vi "APC_9056_StateMachine.vi"(0 "ManualState":i8, 4 "ForceState":bool, 5 "PC_ControlSettings":T1={"Spark advance [CADBTDC]"=0.0, "Pref"=0.0, "O2ref"=0.0, "DI advance [CADBTDC]"=0.0, "DI duration [ms] "=0.0, "CO2ref"=0.0, "PFI duration [ms]"=0.0, "IMEP ref"=0.0, "Speed ref"=0.0, "IGN enable"=TRUE, "DI enable"=TRUE, "CL PFI\n lambda"=TRUE, "CL PFI\nIMEP"=FALSE, "Activate\ncylinder"=[FALSE, FALSE, FALSE, FALSE, FALSE, FALSE], "Force idling"=FALSE, "Force motoring"=FALSE, "ETP resync"=FALSE, "Requested mode"=0, "Clear Sync Errors"=FALSE, "toggle TDC"=FALSE, "l ref"=0.0, "PID control references"={"NG"=FALSE, "Ar"=FALSE, "O2"=FALSE, "Intake vent"=FALSE, "Cross vent"=FALSE, "Exhaust vent"=FALSE, "NG control mode"=0, "NG-FC-001-REF"=0.0, "WF-OA-002-REF"=0.0, "IMEP-REF"=0.0, "Nm-REF"=0.0, "Ar control mode"=0, "AR-PC-002-REF"=0.0, "WF-PT-004-REF"=0.0, "O2 control mode"=0, "O2-FC-001-REF"=0.0, "WF-OA-001-REF"=0.0, "Tcoolant control  mode"=0, "EC-FC-001-REF"=0.0, "EC-TT-001-REF"=0.0, "Texh control mode"=0, "SW-FC-004-REF"=0.0, "SW-FT-002-REF"=0.0, "WF-TT-004-REF"=0.0, "Toil control mode"=0, "SW-FC-009-REF"=0.0, "SW-FT-004-REF"=0.0, "EO-TT-001-REF"=0.0, "AIC201_CO2_ConcTarget"=0.0, "O2_FF_NG"=FALSE, "Dyno control mode"=0, "Membrane control mode"=0, "AR-FT-001-REF"=0.0, "MTR modbus floats"=[0.0, 0.0, 0.0, 0.0, 0.0, 0.0, 0.0, 0.0, 0.0, 0.0, 0.0, 0.0, 0.0, 0.0, 0.0, 0.0, 0.0, 0.0, 0.0], "MTR modbus u16"=[0, 0, 0, 0, 0, 0, 0], "MTR HB"=FALSE, "PC_HB"=FALSE, "EMERGENCY STOP"=FALSE}, "CA50setpoint [CADATDC]"=0.0, "CA50 control"=TRUE, "Knock control"=TRUE, "CLEAR EMERGENCY STOP"=FALSE, "EMERGENCY STOP"=FALSE}, 6 "STATE LIMITATION FROM WARNINGS":i8, 7 "CURRENT SYSTEM STATE":i8) -> (1 "Limited_ControlSettings":T1={"Spark advance [CADBTDC]"=0.0, "Pref"=0.0, "O2ref"=0.0, "DI advance [CADBTDC]"=0.0, "DI duration [ms] "=0.0, "CO2ref"=0.0, "PFI duration [ms]"=0.0, "IMEP ref"=0.0, "Speed ref"=0.0, "IGN enable"=TRUE, "DI enable"=TRUE, "CL PFI\n lambda"=TRUE, "CL PFI\nIMEP"=FALSE, "Activate\ncylinder"=[FALSE, FALSE, FALSE, FALSE, FALSE, FALSE], "Force idling"=FALSE, "Force motoring"=FALSE, "ETP resync"=FALSE, "Requested mode"=0, "Clear Sync Errors"=FALSE, "toggle TDC"=FALSE, "l ref"=0.0, "PID control references"={"NG"=FALSE, "Ar"=FALSE, "O2"=FALSE, "Intake vent"=FALSE, "Cross vent"=FALSE, "Exhaust vent"=FALSE, "NG control mode"=0, "NG-FC-001-REF"=0.0, "WF-OA-002-REF"=0.0, "IMEP-REF"=0.0, "Nm-REF"=0.0, "Ar control mode"=0, "AR-PC-002-REF"=0.0, "WF-PT-004-REF"=0.0, "O2 control mode"=0, "O2-FC-001-REF"=0.0, "WF-OA-001-REF"=0.0, "Tcoolant control  mode"=0, "EC-FC-001-REF"=0.0, "EC-TT-001-REF"=0.0, "Texh control mode"=0, "SW-FC-004-REF"=0.0, "SW-FT-002-REF"=0.0, "WF-TT-004-REF"=0.0, "Toil control mode"=0, "SW-FC-009-REF"=0.0, "SW-FT-004-REF"=0.0, "EO-TT-001-REF"=0.0, "AIC201_CO2_ConcTarget"=0.0, "O2_FF_NG"=FALSE, "Dyno control mode"=0, "Membrane control mode"=0, "AR-FT-001-REF"=0.0, "MTR modbus floats"=[0.0, 0.0, 0.0, 0.0, 0.0, 0.0, 0.0, 0.0, 0.0, 0.0, 0.0, 0.0, 0.0, 0.0, 0.0, 0.0, 0.0, 0.0, 0.0], "MTR modbus u16"=[0, 0, 0, 0, 0, 0, 0], "MTR HB"=FALSE, "PC_HB"=FALSE, "EMERGENCY STOP"=FALSE}, "CA50setpoint [CADATDC]"=0.0, "CA50 control"=TRUE, "Knock control"=TRUE, "CLEAR EMERGENCY STOP"=FALSE, "EMERGENCY STOP"=FALSE}, 3 "SYSTEM STATE":i8)   [LabVIEW 2020]
uses:
  controls/APC_ControlSettings.ctl
  controls/APC_PIDcontrolSettings.ctl
panel:
  out "Aggregate (MIN) State Limitation":i8
  out "STATE LIMITATION FROM Force Idling":i8
  out "STATE LIMITATION FROM Force Motoring":i8
  out "STATE LIMITATION FROM E-STOP":i8
  out "CURRENT SYSTEM STATE":i8
  out "Requested mode":i8
  out "STATE LIMITATION FROM WARNINGS":i8
  in  "DisregardWarnings":bool
  out "maximum controller mode":i32[](array[numeric])
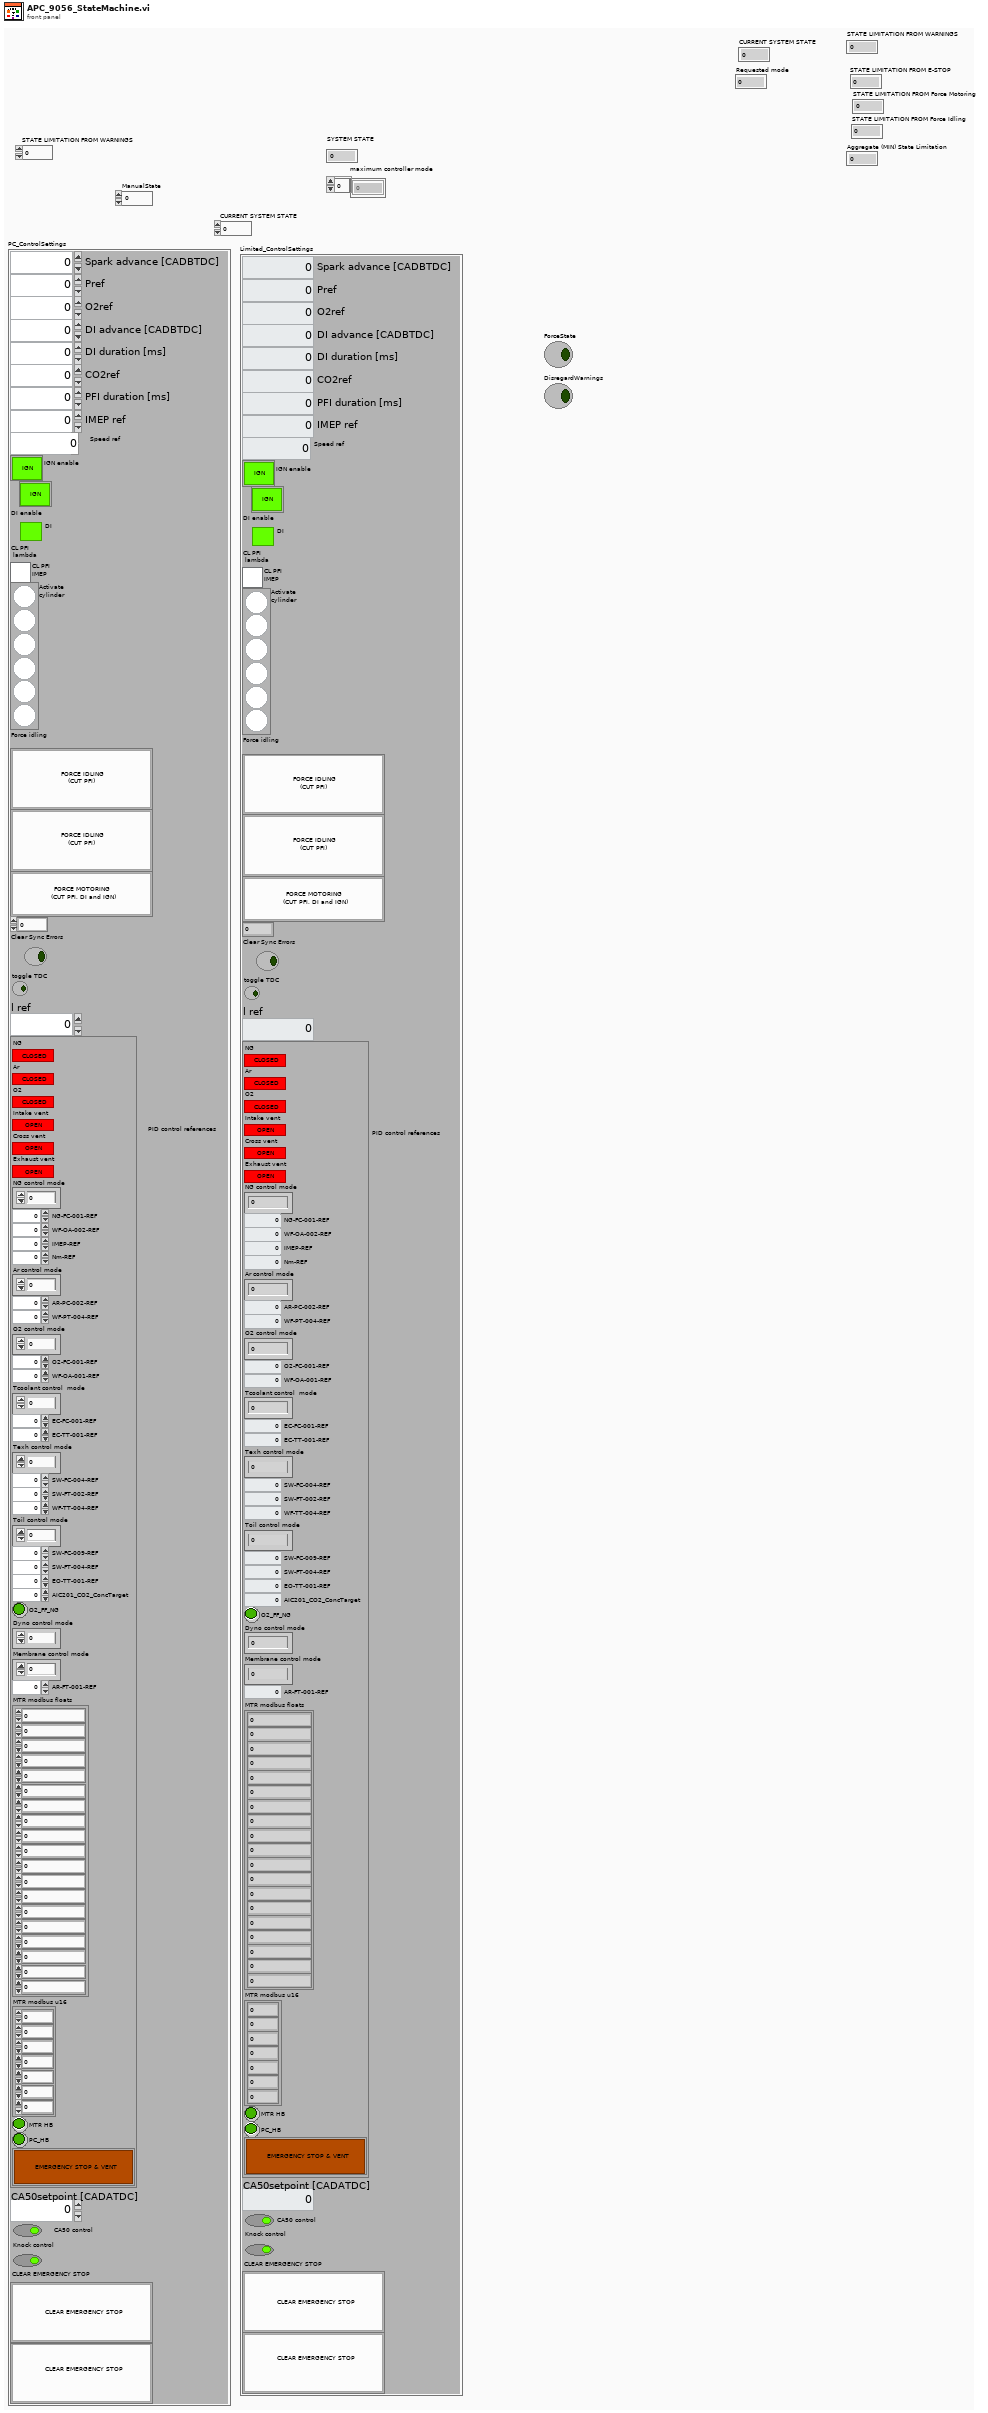
[diagram p1: front panel]
types:
  T1 = typedef "APC_ControlSettings.ctl" = cluster{"Spark advance [CADBTDC]":dbl, "Pref":dbl, "O2ref":dbl, "DI advance [CADBTDC]":dbl, "DI duration [ms] ":dbl, "CO2ref":dbl, "PFI duration [ms]":dbl, "IMEP ref":dbl, "Speed ref":dbl, "IGN enable":bool, "DI enable":bool, "CL PFI\n lambda":bool, "CL PFI\nIMEP":bool, "Activate\ncylinder":bool[], "Force idling":bool, "Force motoring":bool, "ETP resync":bool, "Requested mode":i8, "Clear Sync Errors":bool, "toggle TDC":bool, "l ref":dbl, "PID control references":T2, "CA50setpoint [CADATDC]":dbl, "CA50 control":bool, "Knock control":bool, "CLEAR EMERGENCY STOP":bool, "EMERGENCY STOP":bool}
  T2 = typedef "APC_PIDcontrolSettings.ctl" = cluster{"NG":bool, "Ar":bool, "O2":bool, "Intake vent":bool, "Cross vent":bool, "Exhaust vent":bool, "NG control mode":u8, "NG-FC-001-REF":dbl, "WF-OA-002-REF":dbl, "IMEP-REF":dbl, "Nm-REF":dbl, "Ar control mode":u8, "AR-PC-002-REF":dbl, "WF-PT-004-REF":dbl, "O2 control mode":u8, "O2-FC-001-REF":dbl, "WF-OA-001-REF":dbl, "Tcoolant control  mode":u8, "EC-FC-001-REF":dbl, "EC-TT-001-REF":dbl, "Texh control mode":u8, "SW-FC-004-REF":dbl, "SW-FT-002-REF":dbl, "WF-TT-004-REF":dbl, "Toil control mode":u8, "SW-FC-009-REF":dbl, "SW-FT-004-REF":dbl, "EO-TT-001-REF":dbl, "AIC201_CO2_ConcTarget":dbl, "O2_FF_NG":bool, "Dyno control mode":u8, "Membrane control mode":u8, "AR-FT-001-REF":dbl, "MTR modbus floats":sgl[], "MTR modbus u16":u16[], "MTR HB":bool, "PC_HB":bool, "EMERGENCY STOP":bool}
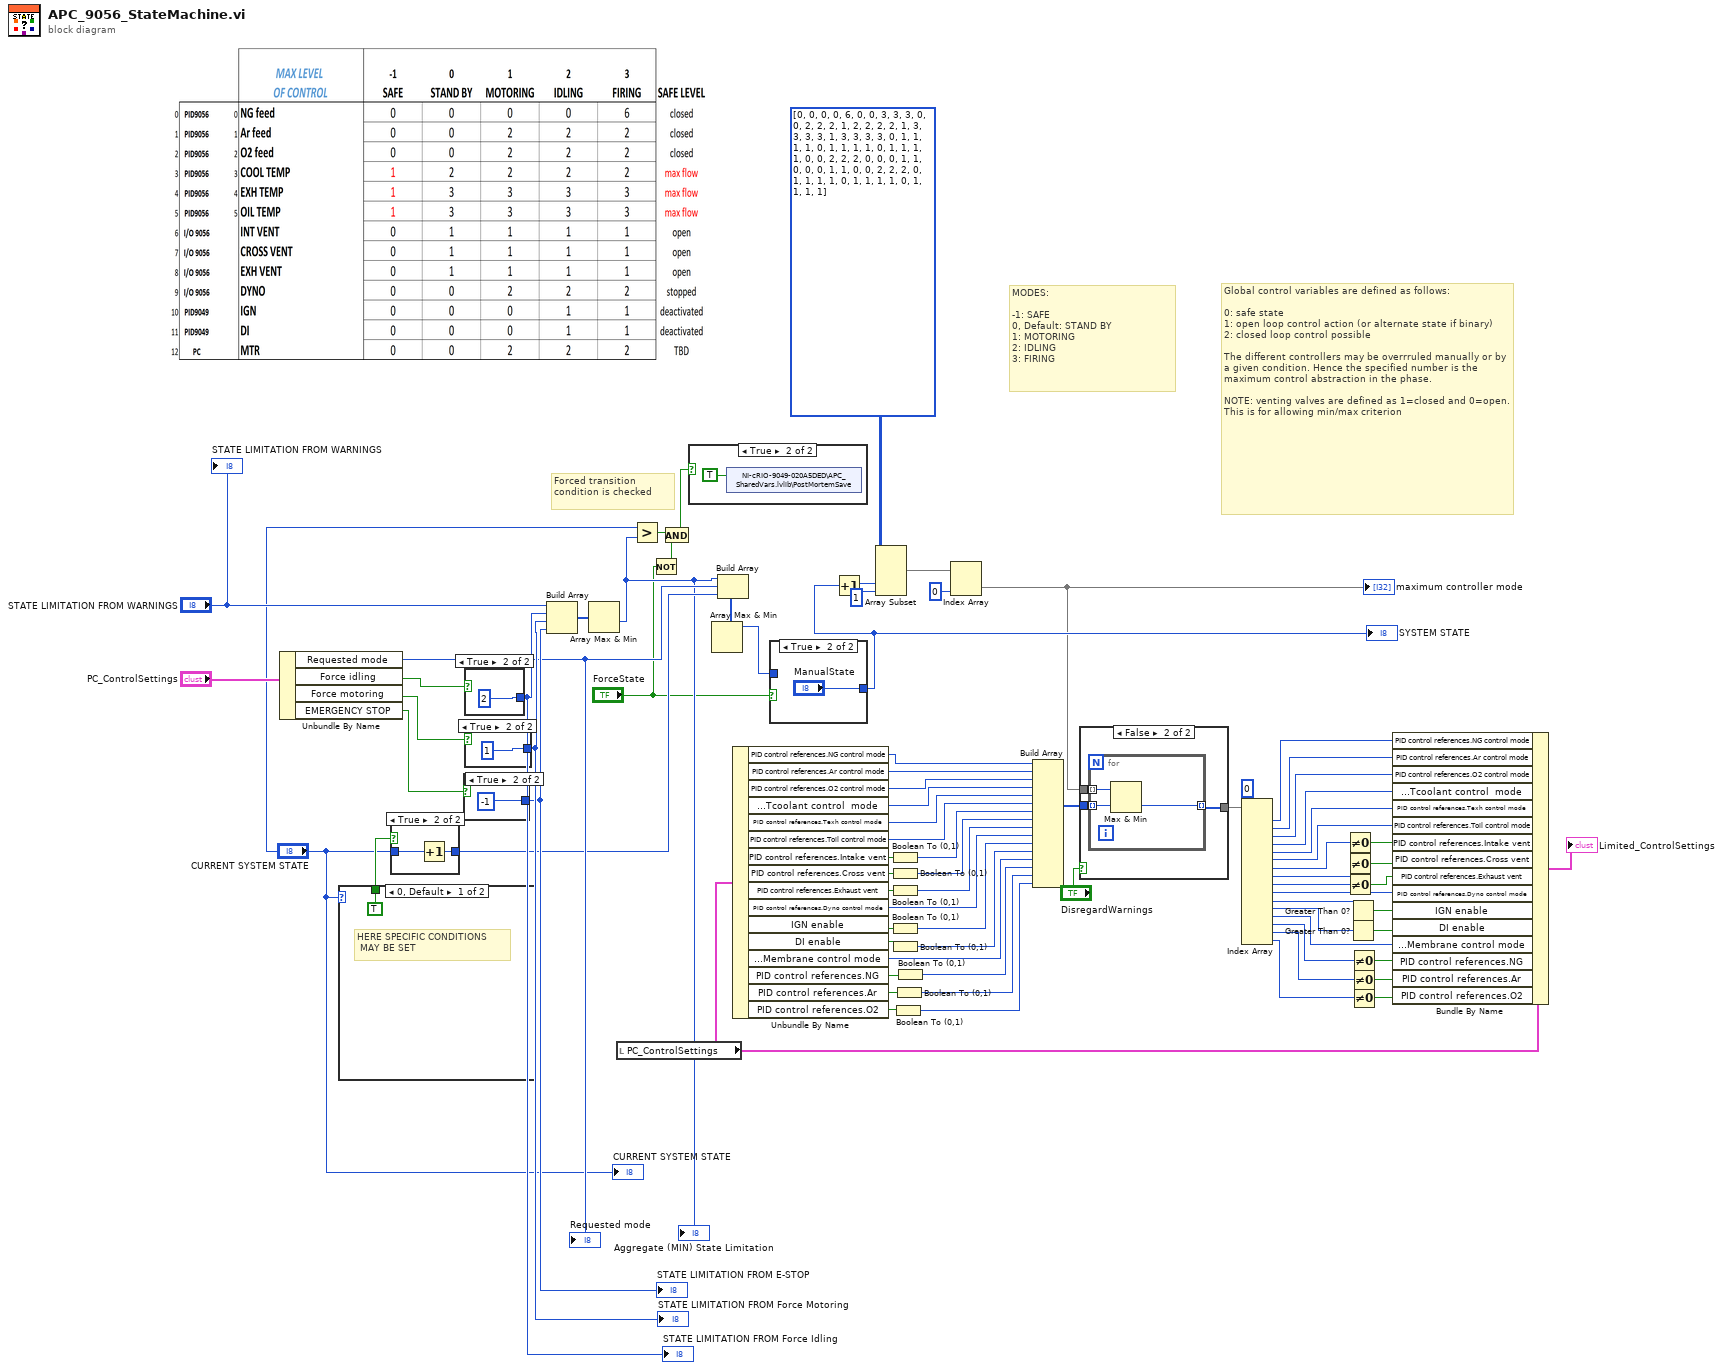
[diagram p0: block diagram]
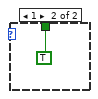
[diagram p6: hidden frame]
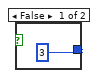
[diagram p7: hidden frame]
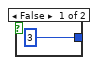
[diagram p8: hidden frame]
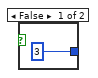
[diagram p9: hidden frame]
diagram:
  # "Forced transition condition is checked"
  # "Global control variables are defined as follows:\n\n0: safe state\n1: open loop control action (or alternate state if binary)\n2: closed loop control possible\n\nThe different controllers may be overrruled manually or by a given condition. Hence the specified number is the maximum control abstraction in the phase.\n\nNOTE: venting valves are defined as 1=closed and 0=open. This is for allowing min/max criterion"
  # "MODES:\n\n-1: SAFE\n0, Default: STAND BY\n1: MOTORING\n2: IDLING\n3: FIRING"
  n1 = Unbundle By Name("PC_ControlSettings") -> ("Requested mode"=w9:i8, "Force idling"=w80:bool, "Force motoring"=w79:bool, "EMERGENCY STOP"=w73:bool)
  "Requested mode" <- w9
  n2 = case shown="0, Default" "CURRENT SYSTEM STATE" {
    tunnel: [TRUE TRUE] -> w75
    frame 0, Default {
      # "HERE SPECIFIC CONDITIONS\n MAY BE SET"
    }
    frame 1 {
    }
  }
  n3 = case shown="True" w75 {
    tunnel: [w84 w86] -> w8
    tunnel: "CURRENT SYSTEM STATE" -> [w84 w85]
    frame False {
    }
    frame True {
      n4 = Increment(x=w85) -> (x+1=w86:i8)
    }
  }
  n5 = case shown="True" w73 {
    tunnel: [i8 3 ("STATE LIMITATION FROM WARNINGS") i8 -1 ("STATE LIMITATION FROM WARNINGS")] -> w74
    frame False {
    }
    frame True {
    }
  }
  "STATE LIMITATION FROM E-STOP" <- w74
  n6 = case shown="True" w80 {
    tunnel: [i8 3 ("STATE LIMITATION FROM WARNINGS") i8 2 ("STATE LIMITATION FROM WARNINGS")] -> w76
    frame False {
    }
    frame True {
    }
  }
  "STATE LIMITATION FROM Force Idling" <- w76
  n7 = case shown="True" w79 {
    tunnel: [i8 3 ("STATE LIMITATION FROM WARNINGS") i8 1 ("STATE LIMITATION FROM WARNINGS")] -> w77
    frame False {
    }
    frame True {
    }
  }
  "STATE LIMITATION FROM Force Motoring" <- w77
  n8 = Build Array("STATE LIMITATION FROM WARNINGS", w76, w77, w74) -> (w78:i8[])
  n9 = Array Max & Min(array=w78) -> (min value=w6:i8)  [unwired: 3 out]
  "Aggregate (MIN) State Limitation" <- w6
  n10 = local read "PC_ControlSettings"() -> (w65:T1)
  n11 = Greater?(x="CURRENT SYSTEM STATE", y=w6) -> (0:w5:bool)
  n12 = Not(x="ForceState") -> (.not. x?=w4:bool)
  n13 = And(x=w5, y=w4) -> (x .and. y?=w2:bool)
  n14 = case shown="True" w2 {
    frame False {
    }
    frame True {
      n15 = shared-variable "NI-cRIO-9049-020A5DED\\APC_SharedVars.lvlib\\PostMortemSave"(TRUE ("PostMortemSave")) -> ()  [unwired: 1 in, 1 out]
    }
  }
  n16 = Build Array(w6, w9, w8) -> (w10:i8[])
  n17 = Array Max & Min(array=w10) -> (min value=w7:i8)  [unwired: 3 out]
  n18 = Unbundle By Name(w65) -> ("PID control references.NG control mode"=w27:u8, "PID control references.Ar control mode"=w28:u8, "PID control references.O2 control mode"=w29:u8, "PID control references.Tcoolant control  mode"=w30:u8, "PID control references.Texh control mode"=w31:u8, "PID control references.Toil control mode"=w32:u8, "PID control references.Intake vent"=w69:bool, "PID control references.Cross vent"=w68:bool, "PID control references.Exhaust vent"=w67:bool, "PID control references.Dyno control mode"=w36:u8, "IGN enable"=w63:bool, "DI enable"=w64:bool, "PID control references.Membrane control mode"=w39:u8, "PID control references.NG"=w26:bool, "PID control references.Ar"=w24:bool, "PID control references.O2"=w22:bool)
  n19 = case shown="True" "ForceState" {
    tunnel: w7 -> [w94 _]
    tunnel: [w94 "ManualState"] -> w41
    frame False {
    }
    frame True {
    }
  }
  "SYSTEM STATE" <- w41
  n20 = Increment(x=w41) -> (x+1=w70:i8)
  n21 = Array Subset(array=i32[][] [[0, 0, 0, 0, 6], [0, 0, 3, 3, 3], [0, 0, 2, 2, 2], [1, 2, 2, 2, 2], [1, 3, 3, 3, 3], [1, 3, 3, 3, 3], [0, 1, 1, 1, 1], [0, 1, 1, 1, 1], [0, 1, 1, 1, 1], [0, 0, 2, 2, 2], [0, 0, 0, 1, 1], [0, 0, 0, 1, 1], [0, 0, 2, 2, 2], [0, 1, 1, 1, 1], [0, 1, 1, 1, 1], [0, 1, 1, 1, 1]], index (col)=w70, length (col)=1 ("length")) -> (w14:i32[][])  [unwired: 2 in]
  n22 = Boolean To (0,1)(Boolean=w69) -> (0, 1=w33:i16)
  n23 = Boolean To (0,1)(Boolean=w68) -> (0, 1=w34:i16)
  n24 = Boolean To (0,1)(Boolean=w67) -> (0, 1=w35:i16)
  n25 = Boolean To (0,1)(Boolean=w63) -> (0, 1=w37:i16)
  n26 = Boolean To (0,1)(Boolean=w64) -> (0, 1=w38:i16)
  n27 = Boolean To (0,1)(Boolean=w22) -> (0, 1=w21:i16)
  n28 = Boolean To (0,1)(Boolean=w24) -> (0, 1=w23:i16)
  n29 = Boolean To (0,1)(Boolean=w26) -> (0, 1=w25:i16)
  n30 = Index Array(array=w14, index (col)=0 ("disabled index (col)")) -> (element=w12:i32[])  [unwired: 1 in]
  "maximum controller mode" <- w12
  n31 = Build Array(w27, w28, w29, w30, w31, w32, w33, w34, w35, w36, w37, w38, w39, w25, w23, w21) -> (w66:i16[])
  n32 = case shown="False" "DisregardWarnings" {
    tunnel: w66 -> [_ w99]
    tunnel: w12 -> [w96 w98]
    tunnel: [w96 w97] -> w62
    frame True {
    }
    frame False {
      n33 = for {
        tunnel: w99 -> [w101] mode=indexing
        tunnel: w98 -> [w102] mode=indexing
        tunnel: [w100] -> w97 mode=indexing
        n34 = Max & Min(x=w102, y=w101) -> (min(x,y)=w100:i32)  [unwired: 1 out]
      }
    }
  }
  n35 = Index Array(array=w62, index #1=0 ("index")) -> (element #1=w60:i32, element #2=w59:i32, element #3=w58:i32, element #4=w57:i32, element #5=w55:i32, element #6=w54:i32, element #7=w48:i32, element #8=w47:i32, element #9=w46:i32, element #10=w45:i32, element #11=w44:i32, element #12=w43:i32, element #13=w42:i32, element #14=w20:i32, element #15=w18:i32, element #16=w16:i32)  [unwired: 15 in]
  n36 = Not Equal To 0?(x=w48) -> (x != 0?=w53:bool)
  n37 = Not Equal To 0?(x=w47) -> (x != 0?=w52:bool)
  n38 = Not Equal To 0?(x=w46) -> (x != 0?=w51:bool)
  n39 = Greater Than 0?(x=w44) -> (x > 0?=w49:bool)
  n40 = Greater Than 0?(x=w43) -> (x > 0?=w50:bool)
  n41 = Not Equal To 0?(x=w20) -> (x != 0?=w19:bool)
  n42 = Not Equal To 0?(x=w18) -> (x != 0?=w17:bool)
  n43 = Not Equal To 0?(x=w16) -> (x != 0?=w15:bool)
  n44 = Bundle By Name(cluster=w65, "PID control references.NG control mode"=w60, "PID control references.Ar control mode"=w59, "PID control references.O2 control mode"=w58, "PID control references.Tcoolant control  mode"=w57, "PID control references.Texh control mode"=w55, "PID control references.Toil control mode"=w54, "PID control references.Intake vent"=w53, "PID control references.Cross vent"=w52, "PID control references.Exhaust vent"=w51, "PID control references.Dyno control mode"=w45, "IGN enable"=w49, "DI enable"=w50, "PID control references.Membrane control mode"=w42, "PID control references.NG"=w19, "PID control references.Ar"=w17, "PID control references.O2"=w15) -> (→"Limited_ControlSettings":T1)
  "STATE LIMITATION FROM WARNINGS" <- "STATE LIMITATION FROM WARNINGS"
  "CURRENT SYSTEM STATE" <- "CURRENT SYSTEM STATE"
